vi "10.2.vi"() -> ()   [LabVIEW 2017]
panel:
  in  "stop":bool caption="press this buton to stop vi :)"
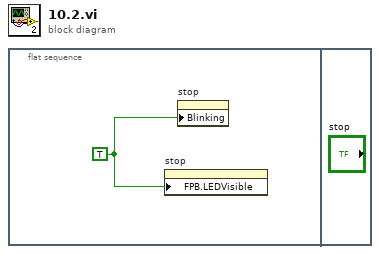
[diagram p0: block diagram]
diagram:
  n1 = flat-sequence {
    frame #0 {
      w1 = TRUE
      n2 = property on="stop" class="Bool"("FPB.LEDVisible"=w1) -> ()  [unwired: 2 in, 2 out]
      n3 = property on="stop" class="Bool"("Blinking"=w1) -> ()  [unwired: 2 in, 2 out]
    }
    frame #1 {
    }
  }
